vi "hw4-6 topVI.vi"() -> ()   [LabVIEW 2014]
panel:
  in  "input file path":path=path "C:/Users/Alvin/Documents/~碩班/Course/109-2/虛擬儀控之設計與應用_吳文中/作業區/HW4/4-6/sample.xml"
  in  "output file path":path
  out "output string":string[](array[string])
  out "input string":string
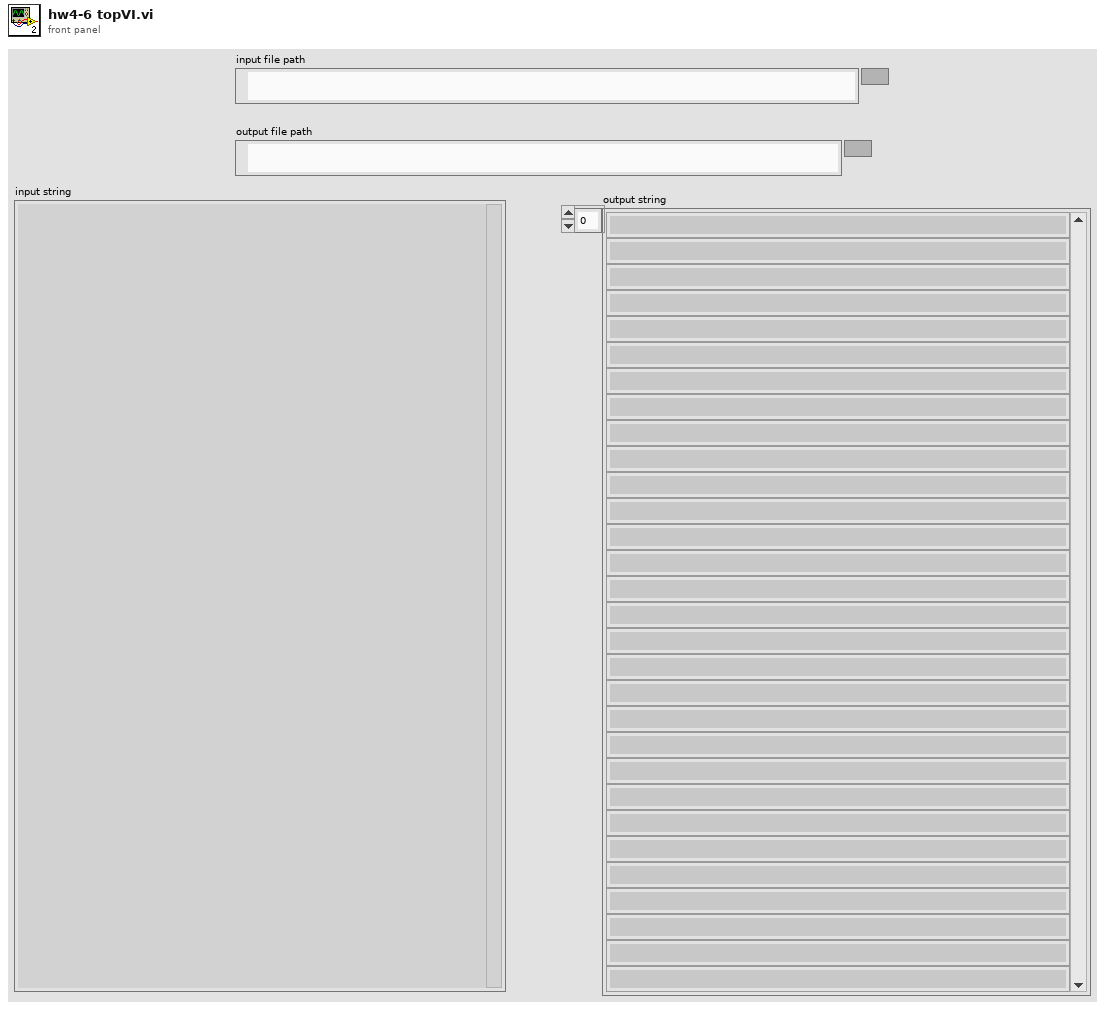
[diagram p1: front panel]
types:
  T1 = enum16{"open", "replace", "create", "open or create", "replace or create", "replace or create with confirmation"}
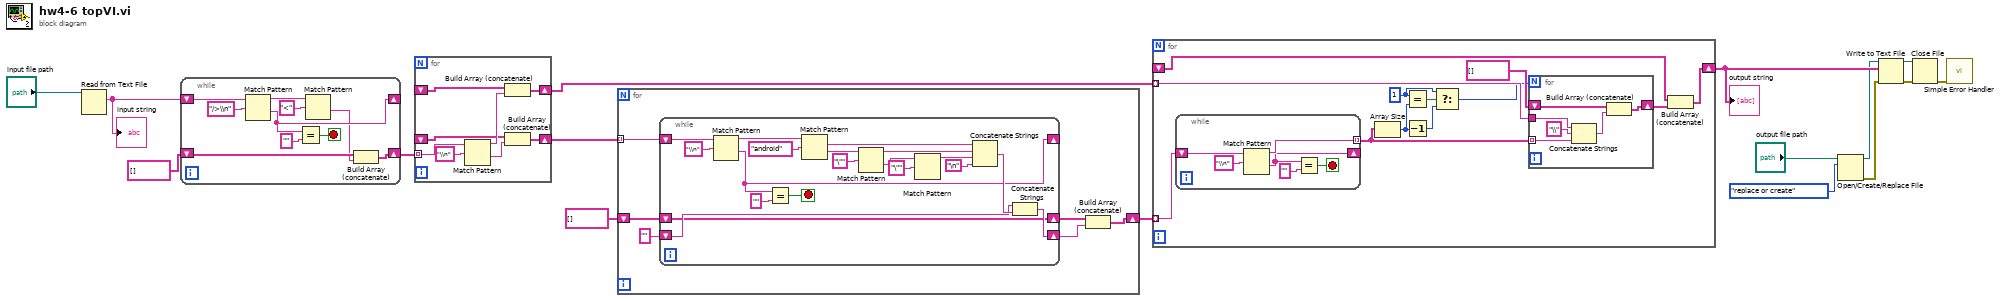
[diagram p0: block diagram]
diagram:
  n1 = Read from Text File(file (use dialog)="input file path") -> (text=w15:string)  [unwired: 3 in, 3 out]
  "input string" <- w15
  n2 = while {
    shift-right: [w20] -> _
    shift-left: w15 -> [w26]
    shift-right: [w22] -> w2
    shift-left: string[] [] -> [w21]
    stop <- w23 stop-if-true
    n3 = Match Pattern(string=w26, regular expression="/>\\n") -> (before substring=w18:string, after substring=w20:string)  [unwired: 1 in, 2 out]
    n4 = Equal?(x=w20, y="") -> (x = y?=w23:bool)
    n5 = Match Pattern(string=w18, regular expression="<") -> (after substring=w19:string)  [unwired: 1 in, 3 out]
    n6 = Build Array (concatenate)(w21, w19) -> (w22:string[])
  }
  n7 = for {
    tunnel: w2 -> [w34] mode=indexing
    shift-right: [w31] -> w1
    shift-left: _ -> [w28]
    shift-right: [w29] -> w13
    shift-left: _ -> [w27]
    n8 = Match Pattern(string=w34, regular expression="\\n") -> (before substring=w32:string, after substring=w30:string)  [unwired: 1 in, 2 out]
    n9 = Build Array (concatenate)(w28, w32) -> (w31:string[])
    n10 = Build Array (concatenate)(w27, w30) -> (w29:string[])
  }
  n11 = for {
    tunnel: w13 -> [w39] mode=indexing
    shift-right: [w37] -> w11
    shift-left: string[] [] -> [w40]
    n12 = while {
      shift-right: [w42] -> _
      shift-left: w39 -> [w50]
      shift-right: [w45] -> w36
      shift-left: w40 -> [w45]
      shift-right: [w47] -> w38
      shift-left: "" -> [w46]
      stop <- w49 stop-if-true
      n13 = Match Pattern(string=w50, regular expression="\\n") -> (before substring=w44:string, after substring=w42:string)  [unwired: 1 in, 2 out]
      n14 = Equal?(x=w42, y="") -> (x = y?=w49:bool)
      n15 = Match Pattern(string=w44, regular expression="android") -> (match substring=w54:string, after substring=w58:string)  [unwired: 1 in, 2 out]
      n16 = Match Pattern(string=w58, regular expression="\"") -> (before substring=w53:string, after substring=w56:string)  [unwired: 1 in, 2 out]
      n17 = Match Pattern(string=w56, regular expression="\"") -> (before substring=w52:string)  [unwired: 1 in, 3 out]
      n18 = Concatenate Strings(w54, w53, w52, "\n") -> (w48:string)
      n19 = Concatenate Strings(w46, w48) -> (w47:string)
    }
    n20 = Build Array (concatenate)(w36, w38) -> (w37:string[])
  }
  n21 = for {
    tunnel: w11 -> [w71] mode=indexing
    tunnel: w1 -> [w70] mode=indexing
    shift-right: [w67] -> w10
    shift-left: _ -> [w66]
    w61 = 1 ("y")
    n22 = while {
      tunnel: [w81] -> w65 mode=indexing
      shift-right: [w79] -> _
      shift-left: w71 -> [w82]
      stop <- w80 stop-if-true
      n23 = Match Pattern(string=w82, regular expression="\\n") -> (before substring=w81:string, after substring=w79:string)  [unwired: 1 in, 2 out]
      n24 = Equal?(x=w79, y="") -> (x = y?=w80:bool)
    }
    n25 = Array Size(array=w65) -> (size(s)=w63:i32)
    n26 = Equal?(x=w61, y=w63) -> (x = y?=w64:bool)
    n27 = Decrement(x=w63) -> (x-1=w62:i32)
    n28 = Select(t=w61, s=w64, f=w62) -> (s? t:f=w60:i32)
    n29 = for {
      N: w60 -> [_]
      tunnel: w65 -> [w77] mode=indexing
      tunnel: w70 -> [w76]
      shift-right: [w73] -> w68
      shift-left: string[] [] -> [w72]
      n30 = Concatenate Strings(w76, "\\" ("string"), w77) -> (w74:string)
      n31 = Build Array (concatenate)(w72, w74) -> (w73:string[])
    }
    n32 = Build Array (concatenate)(w66, w68) -> (w67:string[])
  }
  "output string" <- w10
  n33 = Open/Create/Replace File(file path (use dialog)="output file path", operation (0:open)=T1."replace or create") -> (refnum out=w8:refnum<file>, error out=w7:errorcluster)  [unwired: 4 in, 1 out]
  n34 = Write to Text File(file (use dialog)=w8, text=w10, error in=w7) -> (refnum out=w6:refnum<file>, error out=w5:errorcluster)  [unwired: 1 in, 1 out]
  n35 = Close File(refnum=w6, error in=w5) -> (error out=w4:errorcluster)  [unwired: 1 out]
  n36 = call <vilib>:"Simple Error Handler.vi"("error in (no error)"=w4) -> ()  [unwired: 4 in, 5 out]
